vi "Instrument Configure Call.vi"(0 "VI Refnum":T1, 1 "error in":errorcluster) -> (2 "Numeric":i32, 3 "Stop?":bool, 4 "error out":errorcluster)   [LabVIEW 2020]
uses:
  New NML Data Acq/Sub Controls/Instrument Ref.ctl
  New NML Data Acq/Sub Controls/Instrument Actions.ctl
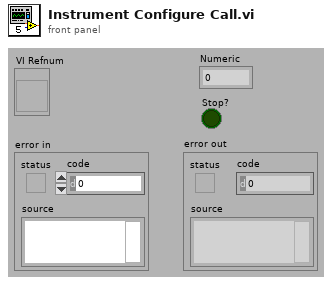
[diagram p1: front panel]
types:
  T1 = typedef "Instrument Ref.ctl" = refnum<vi>
  T2 = typedef "Instrument Actions.ctl" = enum16{"Scan", "Identify", "New", "Configure", "Initialize", "Test", "Read", "Close"}
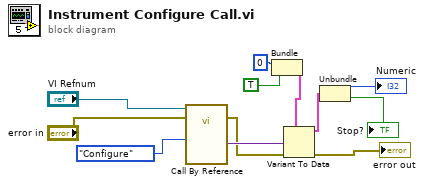
[diagram p0: block diagram]
diagram:
  n1 = call-by-ref "?"(reference="VI Refnum", error in="error in", "Action"=Instrument_Actions."Configure") -> (error out=w8:errorcluster, "Output"=w10:variant)  [unwired: 5 in, 2 out]
  n2 = Bundle(0, TRUE) -> (w6:cluster{i32, bool})  [unwired: 1 in]
  n3 = Variant To Data(error in=w8, type=w6, Variant=w10) -> (data=w12:cluster{i32, bool}, error out=→"error out":errorcluster)
  n4 = Unbundle(w12) -> (→"Numeric":i32, →"Stop?":bool)
